vi "Disconnect.vi"(8 "error in (no error)":errorcluster, 11 "N5745A in":refnum<class "5745A.lvclass">) -> (0 "error out":errorcluster, 3 "N5745A out":refnum<class "5745A.lvclass">)   [LabVIEW 2018, in "5745A.lvlib" / "5745A.lvclass"]
doc: "This Override method closes communication with the N5745A instrument."
uses:
  5745A.lvclass
  builds/Power_Supply.lvlibp/Power Supply.lvclass
  C:/Users/Ron.Dexter.LUMINARTECH/Desktop/builds/Power_Supply.lvlibp/Power Supply.lvclass
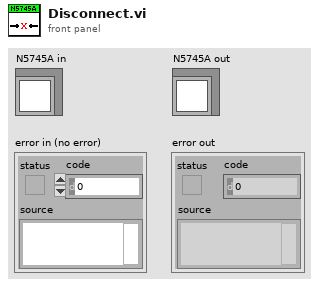
[diagram p1: front panel]
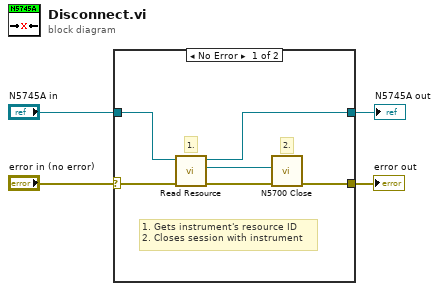
[diagram p0: block diagram]
diagram:
  n1 = case shown="No Error" "error in (no error)" {
    selector: "error in (no error)" -> [w7 w11]
    tunnel: "N5745A in" -> [w6 w12]
    tunnel: [w5 w12] -> w3
    tunnel: [w8 w11] -> w2
    frame No Error {
      # "1. Gets instrument's resource ID\n2. Closes session with instrument"
      # "2."
      # "1."
      n2 = call "Read Resource.vi"("error in"=w7, "Power Supply in"=w6) -> ("error out"=w9:errorcluster, "Resource"=w10:refnum<visa-resource-name>, "Power Supply out"=w5:refnum<class "5745A.lvclass">)  [unwired: 7 in]
      n3 = call <instrlib>:"N5700 Close.vi"("error"=w9, "VISA name"=w10) -> ("error out"=w8:errorcluster)  [unwired: 6 in]
    }
    frame Error {
    }
  }
  "error out" <- w2
  "N5745A out" <- w3
